vi "34970A Config Leak Pressure Read.vi"(4 "Advanced Config":T1={"Aperture Value (.4)"=0.4, "Aperture (1:Minimum)"=enum."Minimum", "NPLC (1)"=enum."2", "Bandwidth (3 Hz)"=enum."3 Hz", "Input Impedance (F:Fixed)"=FALSE, "Integration Time (F:Aperture)"=TRUE} {"Aperture Value (.4)" min=0.4 max=4.0 format="%.2f"}, 5 "Press Scaling":T3(array[cluster])=[{"Gain"=7.5, "Offset"=-7.5, "Units"="PSI", "Channel"="101", "Name"="Fill 1"}, {"Gain"=7.5, "Offset"=-7.5, "Units"="PSI", "Channel"="102", "Name"="Ref 1"}, {"Gain"=2.0, "Offset"=-0.038, "Units"="H2O", "Channel"="103", "Name"="Diff 1"}, {"Gain"=7.5, "Offset"=7.5, "Units"="PSI", "Channel"="104", "Name"="Fill 2"}, {"Gain"=7.5, "Offset"=-7.46, "Units"="PSI", "Channel"="105", "Name"="Ref 2"}, {"Gain"=2.0, "Offset"=0.0, "Units"="H2O", "Channel"="106", "Name"="Diff 2"}], 6 "error in":errorcluster, 7 "Voltage Range (6:Max)":T2(ring)=enum."10 V", 8 "DC/AC (F:DC)":bool, 9 "VISA session":refnum<visa-resource-name>) -> (0 "error out":errorcluster, 2 "#channels":i32, 3 "VISA resource name out":refnum<visa-resource-name>)   [LabVIEW 2020]
panel:
  # "Auto\nFixed"
  # "NPLC\nAperture"
  # "Don't change name or channel"
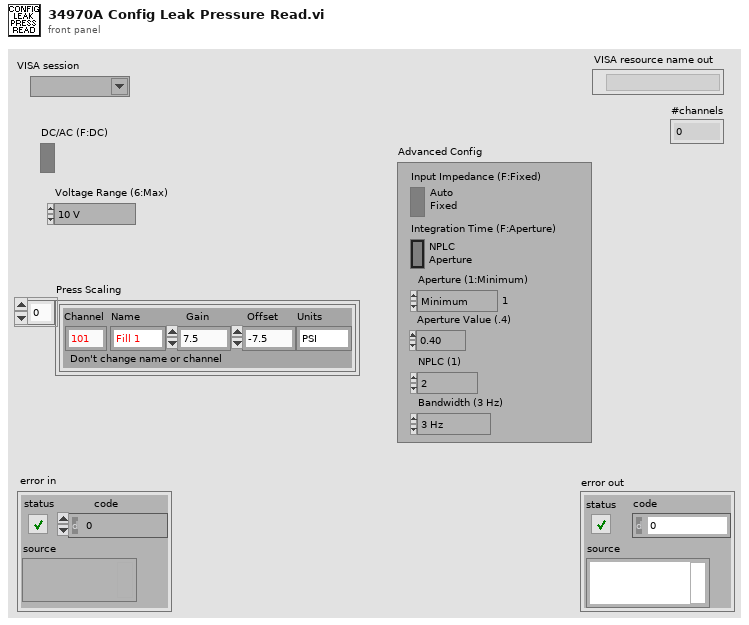
[diagram p1: front panel]
types:
  T1 = cluster{"Aperture Value (.4)":dbl, "Aperture (1:Minimum)":enum16{"Manual", "Minimum", "Maximum"}, "NPLC (1)":enum16{".02", ".2", "1", "2", "10", "20", "100", "200", "Minimum", "Maximum"}, "Bandwidth (3 Hz)":enum16{"3 Hz", "20 Hz", "200 Hz", "Minimum", "Maximum"}, "Input Impedance (F:Fixed)":bool, "Integration Time (F:Aperture)":bool}
  T2 = enum16{"100 mV", "1 V", "10 V", "100 V", "300 V", "Minimum", "Maximum"}
  T3 = cluster{"Gain":dbl, "Offset":dbl, "Units":string, "Channel":string, "Name":string}[]
  T4 = enum16{"Manual", "Minimum", "Maximum", "Infinity"}
  T5 = enum16{"Bus", "Immediate", "External", "Alarm 1", "Alarm 2", "Alarm 3", "Alarm 4", "Timer"}
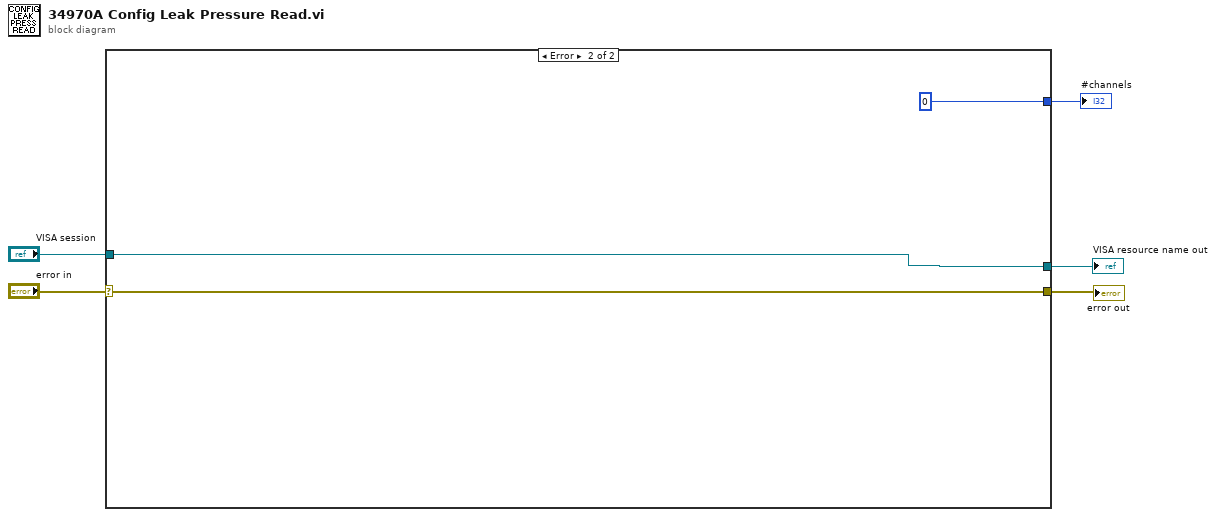
[diagram p0: block diagram]
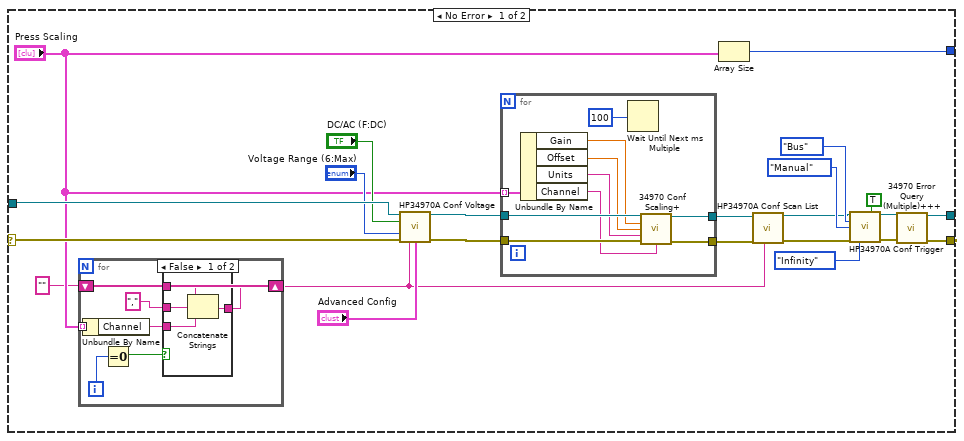
[diagram p2: hidden frame]
diagram:
  n1 = case shown="Error" "error in" {
    selector: "error in" -> [w17 w52]
    tunnel: "VISA session" -> [w28 w53]
    tunnel: [w22 w53] -> w4
    tunnel: [w21 w52] -> w3
    tunnel: [w18 0] -> w2
    frame No Error {
      n2 = for {
        tunnel: "Press Scaling" -> [w35] mode=indexing
        shift-right: [w31] -> w6
        shift-left: "" ("Channel") -> [w30]
        i -> [w34]
        n3 = Unbundle By Name(w35) -> ("Channel"=w32:string)
        n4 = Equal To 0?(x=w34) -> (x = 0?=w33:bool)
        n5 = case shown="False" w33 {
          tunnel: [w36 w40] -> w31
          tunnel: w32 -> [w37 w40]
          tunnel: w30 -> [w39 _]
          tunnel: "," ("string") -> [w38 _]
          frame False {
            n6 = Concatenate Strings(w39, w38, w37) -> (w36:string)
          }
          frame True {
          }
        }
      }
      n7 = call "HP34970A Conf Voltage.vi"("VISA session"=w28, "DC/AC (F:DC)"="DC/AC (F:DC)", "Voltage Range (6:Max)"="Voltage Range (6:Max)", "error in (no error)"=w17, "Channel List(empty)"=w6, "Advanced Config (F/1/4/1/3)"="Advanced Config") -> ("dup VISA session"=w24:refnum<visa-resource-name>, "error out"=w23:errorcluster)  [unwired: 7 in, 1 out]
      n8 = for {
        tunnel: [w50] -> w20
        tunnel: [w49] -> w19
        tunnel: w24 -> [w47]
        tunnel: w23 -> [w46]
        tunnel: "Press Scaling" -> [w45] mode=indexing
        n9 = Unbundle By Name(w45) -> ("Gain"=w41:dbl, "Offset"=w42:dbl, "Units"=w43:string, "Channel"=w44:string)
        n10 = Wait Until Next ms Multiple(millisecond multiple=u32 100) -> ()  [unwired: 1 out]
        n11 = call "34970 Conf Scaling+.vi"("VISA session"=w47, "Gain (1)"=w41, "Offset (0)"=w42, "Units(empty)"=w43, "error in (no error)"=w46, "Channel List(empty)"=w44) -> ("dup VISA session"=w50:refnum<visa-resource-name>, "error out"=w49:errorcluster)  [unwired: 7 in, 1 out]
      }
      n12 = Array Size(array="Press Scaling") -> (size(s)=w18:i32)
      n13 = call "HP34970A Conf Scan List.vi"("Scan List(empty)"=w6, "error in (no error)"=w19, "VISA session"=w20) -> ("error out"=w12:errorcluster, "dup VISA session"=w11:refnum<visa-resource-name>)  [unwired: 6 in, 1 out]
      n14 = call "HP34970A Conf Trigger.vi"("VISA session"=w11, "Wait for Trigger? (F:No)"=TRUE, "Source (1:Immediate)"=T5."Bus", "Scan-Scan Interval (1:Min)"=enum16{"Manual", "Minimum", "Maximum"}."Manual", "error in (no error)"=w12, "Max Trigger Count (3:Inf)"=T4."Infinity") -> ("dup VISA session"=w10:refnum<visa-resource-name>, "error out"=w9:errorcluster)  [unwired: 7 in, 1 out]
      n15 = call "34970 Error Query (Multiple)+++.vi"("VISA resource name"=w10, "error in (no error)"=w9) -> ("VISA resource name out"=w22:refnum<visa-resource-name>, "error out"=w21:errorcluster)  [unwired: 10 in, 2 out]
    }
    frame Error {
    }
  }
  "VISA resource name out" <- w4
  "error out" <- w3
  "#channels" <- w2
